vi "Queue Number Check.vi"() -> ()   [LabVIEW 2020]
panel:
  out "Quit":bool=TRUE
  in  "Data List":i32(listbox)
  in  "Count Time":u32=1000
  out "Count":u32
  out "Read Delay":u32(graph)
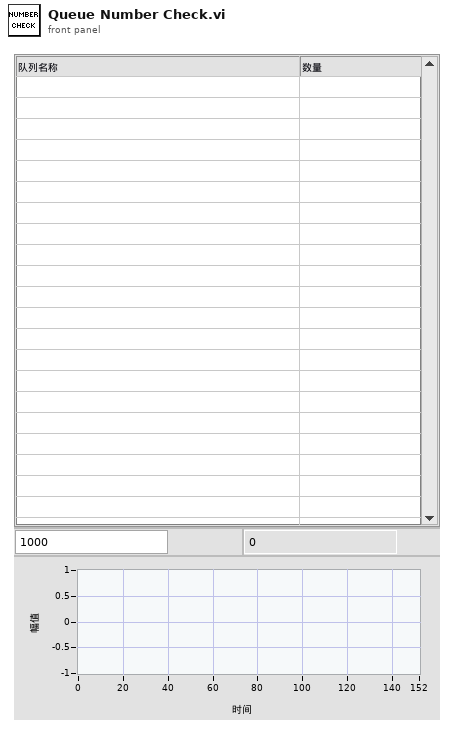
[diagram p1: front panel]
types:
  T1 = enum32{"invalid app kind", "Development System", "Run Time System", "Student Edition", "Embedded LabVIEW", "Evaluation", "Custom"}
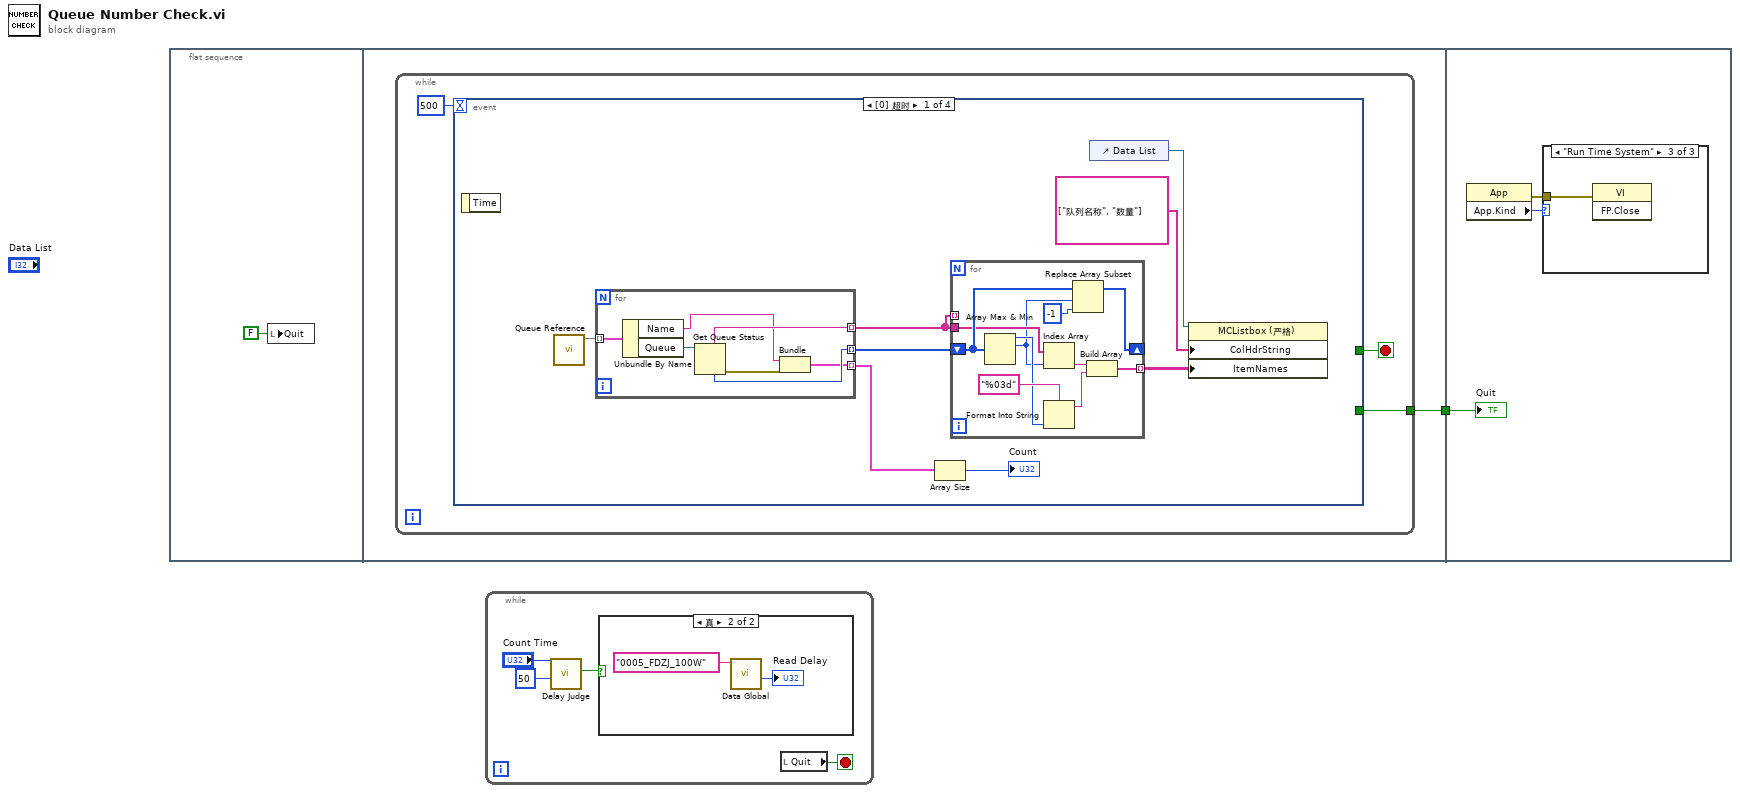
[diagram p0: block diagram]
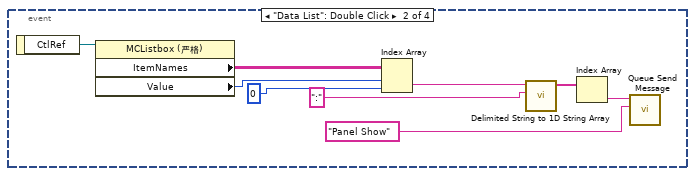
[diagram p3: hidden frame]
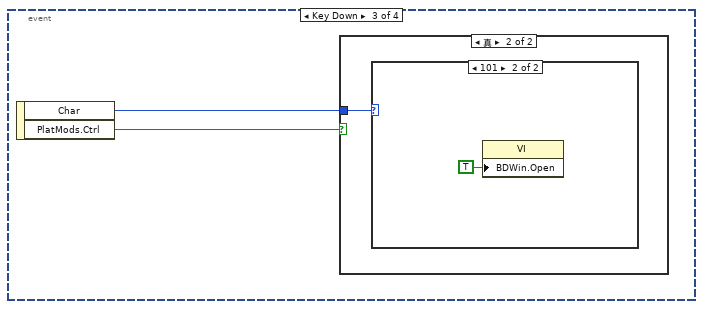
[diagram p4: hidden frame]
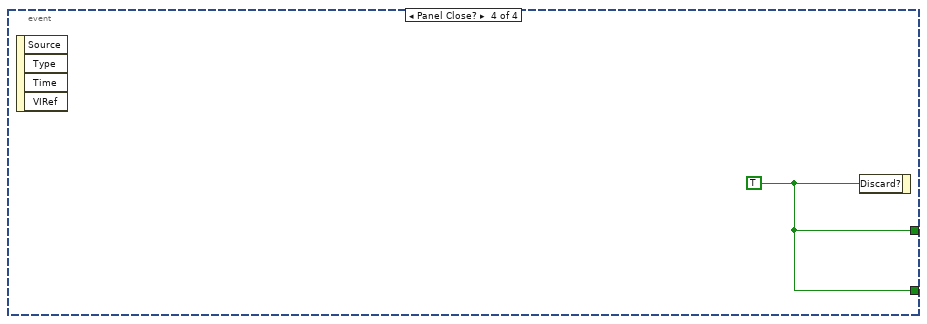
[diagram p7: hidden frame]
diagram:
  n1 = flat-sequence {
    tunnel: [w3] -> w1
    tunnel: w1 -> [w46]
    frame #0 {
      n2 = local write "Quit"(FALSE ("Quit")) -> ()
    }
    frame #1 {
      n3 = while {
        tunnel: [w4] -> w3
        stop <- w6 stop-if-true
        n4 = event shown="[0] 超时" {
          selector: _ -> [_ _ _ _]
          dyn-events: _ -> [_ _ _ _]
          timeout: 500 -> [_ _ _ _]
          tunnel: [_ _ _ w45] -> w6
          tunnel: [_ _ _ w45] -> w4
          event Timeout {
            n5 = event-data() -> ()  [unwired: 1 in, 1 out]
            n6 = call "Queue Reference.vi"() -> ("All Queue"=w10:map{string, refnum<queue>})  [unwired: 8 in, 3 out]
            n7 = for {
              tunnel: w10 -> [w31] mode=indexing
              tunnel: [w29] -> w13 mode=indexing
              tunnel: [w28] -> w12 mode=indexing
              tunnel: [w25] -> w8 mode=indexing
              n8 = Unbundle By Name(w31) -> ("Name"=w26:string, "Queue"=w30:refnum<queue>)
              n9 = Get Queue Status(queue=w30) -> (queue name=w29:string, error out=w27:errorcluster, # elements in queue=w28:i32)  [unwired: 2 in, 5 out]
              n10 = Bundle("Name"=w26, "error out"=w27) -> (w25:cluster{"Name":string, "error out":errorcluster})  [unwired: 1 in]
            }
            n11 = Array Size(array=w8) -> (size(s)=→"Count":i32)
            n12 = for {
              shift-right: [w23] -> _
              shift-left: w12 -> [w24]
              tunnel: w13 -> [w22]
              tunnel: w13 -> [_] mode=indexing
              tunnel: [w15] -> w14 mode=indexing
              n13 = Array Max & Min(array=w24) -> (max value=w20:i32, max index (indices)=w17:i32)  [unwired: 2 out]
              n14 = Index Array(array=w22, index=w17) -> (element=w19:string)
              n15 = Format Into String(format string="%03d" ("格式字符串"), w20) -> (resulting string=w18:string)  [unwired: 2 in, 1 out]
              n16 = Replace Array Subset(array=w24, new element=-1 ("新元素/子数组"), index=w17) -> (w23:i32[])
              n17 = Build Array(w19, w18) -> (w15:string[])
            }
            n18 = control-ref of="Data List"() -> (w11:refnum<vi>)
            n19 = property class="MCListbox (严格)"(reference=w11, "ColHdrString"=string[] ["队列名称", "数量"] ("列首字符串[]"), "ItemNames"=w14) -> ()  [unwired: 1 in, 2 out]
          }
          event "Data List": Double Click {
            n20 = event-data() -> ("CtlRef"=w40:refnum<vi>)  [unwired: 1 in]
            n21 = property class="MCListbox (严格)"(reference=w40) -> ("ItemNames"=w39:string[][], "Value"=w38:i32)  [unwired: 1 in, 2 out]
            n22 = Index Array(array=w39, index (row)=w38, index (col)=0 ("禁用的索引 (列)")) -> (element=w36:string)
            n23 = call <vilib>:"Delimited String to 1D String Array.vi"("delimiter"=":", "delimited string"=w36) -> ("string array"=w34:string[])  [unwired: 9 in]
            n24 = Index Array(array=w34) -> (element=w33:string)  [unwired: 1 in]
            n25 = call "Queue Send Message.vi"("Message"="Panel Show", "Queue Name"=w33) -> ()  [unwired: 7 in, 3 out]
          }
          event Key Down {
            n26 = event-data() -> ("Char"=w42:i16, "PlatMods.Ctrl"=w41:bool)  [unwired: 1 in]
            n27 = case shown="真" w41 {
              tunnel: w42 -> [_ w43]
              frame False {
              }
              frame True {
                n28 = case shown="101" w43 {
                  frame 0, Default {
                  }
                  frame 101 {
                    n29 = property class="VI"("BDWin.Open"=TRUE ("程序框图窗口:打开")) -> ()  [unwired: 2 in, 2 out]
                  }
                }
              }
            }
          }
          event Panel Close? {
            w45 = TRUE ("放弃？")
            n30 = event-data() -> ()  [unwired: 1 in, 4 out]
            n31 = event-data("Discard?"=w45) -> ()  [unwired: 1 in, 1 out]
          }
        }
      }
    }
    frame #2 {
      n32 = property class="App"() -> (error out=w47:errorcluster, "App.Kind"=w48:T1)  [unwired: 2 in, 1 out]
      n33 = case shown="\"Run Time System\"" w48 {
        tunnel: w47 -> [_ _ w49]
        frame "invalid app kind", Default {
        }
        frame "Development System" {
        }
        frame "Run Time System" {
          n34 = invoke class="VI" method="FP.Close"(error in=w49) -> ()  [unwired: 2 in, 3 out]
        }
      }
      "Quit" <- w46
    }
  }
  n35 = while {
    stop <- w51 stop-if-true
    n36 = call "Delay Judge.vi"("Delay Time(ms)"=u32 50, "Count Time(ms)"="Count Time") -> ("Time Out?"=w50:bool)  [unwired: 5 in, 4 out]
    n37 = case shown="真" w50 {
      frame False {
      }
      frame True {
        n38 = call "Data Global.vi"("Name"="0005_FDZJ_100W") -> ("x-y"=→"Read Delay":u32)  [unwired: 7 in, 3 out]
      }
    }
    n39 = local read "Quit"() -> (w51:bool)
  }
